vi "TWM Client Version.vi"() -> (0 "version string":string="1.9.3.0")   [LabVIEW 2020, in "TWM Client.lvlib"]
doc: "This is just a holding VI for TWM client version. Do not edit. It is set programatically when making a build!"
uses:
  TWM Client.lvlib
panel:
  # "this comes from build spec automaticaly!"
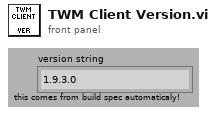
[diagram p1: front panel]
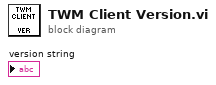
[diagram p0: block diagram]
diagram:
